vi "Read Tare Settings.vi"(7 "Unit ID (A)":string="A", 8 "error in":errorcluster, 11 "VISA Session In":refnum<visa-resource-name>="Alicat") -> (0 "error out":errorcluster, 2 "Tare Functions":T1={"Display"=enum."None", "External"=enum."None", "Auto-Tare Delay [s]"=nan} {"Auto-Tare Delay [s]" format="%.1g"}, 3 "VISA Session Out":refnum<visa-resource-name>)   [LabVIEW 2020]
doc: "Returns the tare settings of an Alicat device: Which variable the display tare button is for, Which variable the remote tare pin is associated with, and the auto tare delay upon power up (0 indicates no tare upon power up)."
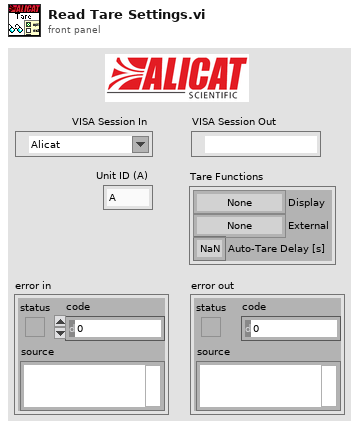
[diagram p1: front panel]
types:
  T1 = cluster{"Display":enum16{"None", "Pressure", "Volumetric"}, "External":enum16{"None", "Pressure", "Volumetric", "Totalizer"}, "Auto-Tare Delay [s]":dbl}
  T2 = cluster{"Display":enum16{"None", "Pressure", "Volumetric"}, "External":enum16{"None", "Pressure", "Volumetric", "Totalizer"}, "Auto Tare Delay":dbl}
  T3 = enum16{"None", "Pressure", "Volumetric", "Totalizer"}
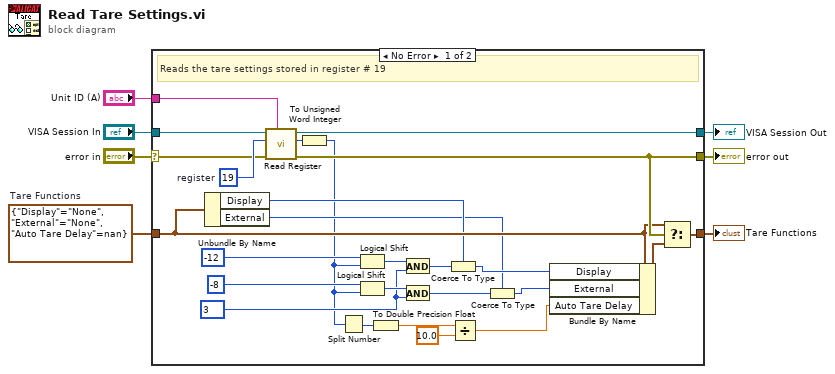
[diagram p0: block diagram]
diagram:
  w3 = T2 {"Display"=enum."None", "External"=enum."None", "Auto Tare Delay"=nan}  # Tare Functions
  n1 = case shown="No Error" "error in" {
    selector: "error in" -> [w8 w35]
    tunnel: "VISA Session In" -> [w32 w36]
    tunnel: "Unit ID (A)" -> [w31 _]
    tunnel: [w30 w36] -> w5
    tunnel: [w29 w35] -> w4
    tunnel: w3 -> [w23 w34]
    tunnel: [w17 w34] -> w2
    frame No Error {
      w22 = u16 3 ("mask")
      w33 = u16 19  # register
      # "Reads the tare settings stored in register # 19"
      n2 = Unbundle By Name(w23) -> ("Display"=w15:enum16{"None", "Pressure", "Volumetric"}, "External"=w12:T3)
      n3 = call "Read Register.vi"("Unit ID (A)"=w31, "error in"=w8, "Register address"=w33, "VISA Session In"=w32) -> ("error out"=w29:errorcluster, "Register Value (I32)"=w10:i32, "VISA Session Out"=w30:refnum<visa-resource-name>)  [unwired: 5 in]
      n4 = To Unsigned Word Integer(number=w10) -> (unsigned 16bit integer=w9:u16)
      n5 = Split Number(x=w9) -> (lo(x)=w21:u8)  [unwired: 1 out]
      n6 = Logical Shift(y=i8 -12, x=w9) -> (x << y=w27:u16)
      n7 = Logical Shift(y=i8 -8, x=w9) -> (x << y=w26:u16)
      n8 = To Double Precision Float(number=w21) -> (double precision float=w19:dbl)
      n9 = And(x=w27, y=w22) -> (x .and. y?=w16:u16)
      n10 = And(x=w26, y=w22) -> (x .and. y?=w13:u16)
      n11 = Coerce To Type(0:w16, 1:w15) -> (2:w14:enum16{"None", "Pressure", "Volumetric"})
      n12 = Divide(x=w19, y=10.0) -> (x/y=w18:dbl)
      n13 = Coerce To Type(0:w13, 1:w12) -> (2:w11:T3)
      n14 = Bundle By Name(cluster=w23, "Display"=w14, "External"=w11, "Auto Tare Delay"=w18) -> (w24:T2)
      n15 = Select(t=w23, s=w29, f=w24) -> (s? t:f=w17:T2)
    }
    frame Error {
    }
  }
  "error out" <- w4
  "VISA Session Out" <- w5
  "Tare Functions" <- w2
